vi "20211225 vision-1 main.vi"(8 "error in":errorcluster) -> (0 "error out":errorcluster, 3 "position":dbl)   [LabVIEW 2019]
panel:
  out "Array":dbl[](array[numeric])
  out "Image Out":T1(plugin-control)
  out "subarray":dbl[](array[numeric])
  in  "Stop (F)":bool
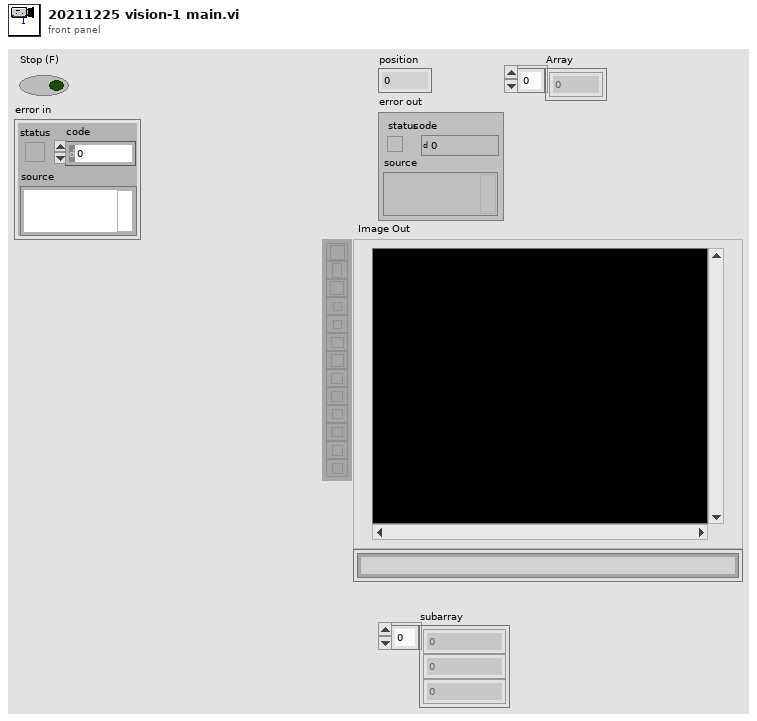
[diagram p1: front panel]
types:
  T1 = typedef "IMAQ Image.ctl" = refnum<image>
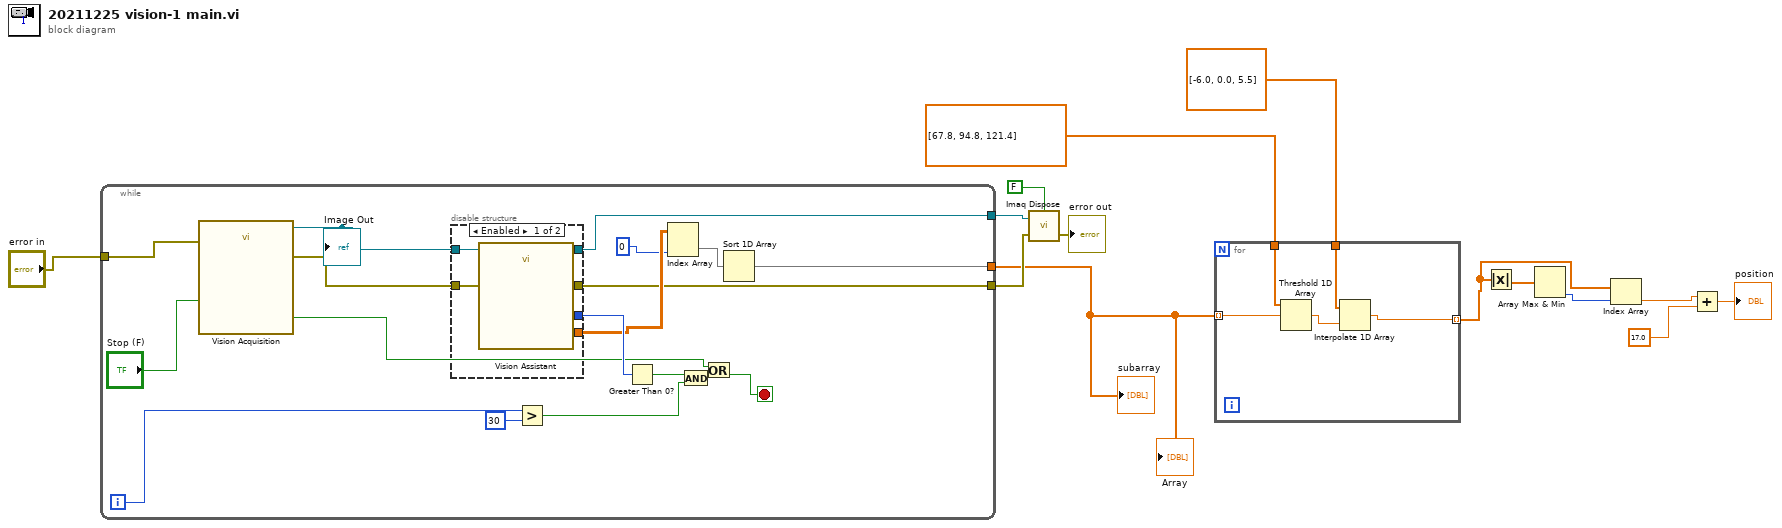
[diagram p0: block diagram]
diagram:
  n1 = while {
    tunnel: [w23] -> w14
    tunnel: [w22] -> w13
    tunnel: [w20] -> w10
    tunnel: "error in" -> [w19]
    i -> [w17]
    stop <- w27 stop-if-true
    n2 = call "Vision Acquisition"("Stop (F)"="Stop (F)", "error in"=w19) -> ("Image Out"=w30:T1, "Stopped"=w26:bool, "error out"=w31:errorcluster)  [unwired: 23 in]
    "Image Out" <- w30
    n3 = disable-structure shown="Enabled" {
      disable-tunnel: w31 -> [w38 _]
      disable-tunnel: w30 -> [w37 _]
      disable-tunnel: [w36 _] -> w29
      disable-tunnel: [w35 _] -> w25
      disable-tunnel: [w34 _] -> w23
      disable-tunnel: [w33 _] -> w22
      frame Enabled {
        n4 = call "Vision Assistant"("Image In"=w37, "error in"=w38) -> ("Image Out"=w34:T1, "Number of Particles (Particle Analysis 1)"=w36:i32, "Particle Measurements (Pixels) (Particle Analysis 1)"=w35:dbl[][], "error out"=w33:errorcluster)  [unwired: 21 in, 1 out]
      }
      frame Disabled {
      }
    }
    n5 = Greater?(x=w17, y=30) -> (0:w15:bool)
    n6 = Greater Than 0?(x=w29) -> (x > 0?=w28:bool)
    n7 = Index Array(array=w25, index (col)=0 ("index (row)")) -> (element=w21:dbl[])  [unwired: 1 in]
    n8 = And(x=w28, y=w15) -> (x .and. y?=w18:bool)
    n9 = Or(x=w26, y=w18) -> (x .or. y?=w27:bool)
    n10 = Sort 1D Array(array=w21) -> (sorted array=w20:dbl[])
  }
  "subarray" <- w10
  "Array" <- w10
  n11 = call "Imaq Dispose"("All Images? (No)"=FALSE, "Image"=w14, "error in (no error)"=w13) -> ("error out"=→"error out":errorcluster)  [unwired: 3 in]
  n12 = for {
    tunnel: dbl[] [67.8, 94.8, 121.4] ("subarray") -> [w43]
    tunnel: w10 -> [w42] mode=indexing
    tunnel: dbl[] [-6.0, 0.0, 5.5] ("array of numbers or points") -> [w40]
    tunnel: [w39] -> w7 mode=indexing
    n13 = Threshold 1D Array(2:w42, 3:w43) -> (0:w41:dbl)  [unwired: 1 in]
    n14 = Interpolate 1D Array(1:w41, 2:w40) -> (0:w39:dbl)
  }
  n15 = Absolute Value(x=w7) -> (abs(x)=w8:dbl[])
  n16 = Array Max & Min(array=w8) -> (min index (indices)=w6:i32)  [unwired: 3 out]
  n17 = Index Array(array=w7, index=w6) -> (element=w5:dbl)
  n18 = Add(x=w5, y=17.0) -> (x+y=→"position":dbl)
